vi "Execute.vi"(0 "Session Handle in":T1, 11 "error in (no error)":errorcluster) -> (4 "Session Handle out":T1, 15 "error out":errorcluster)   [LabVIEW 2020, in "TSS.lvlib" / "Execution.lvclass"]
uses:
  Execution.lvclass
  Typedefs/Session Handle.ctl
  Execution.lvclass/Execution.ctl
  VariableContainer/Get Ref Prop.vi
  SequenceFile/Get Ref Prop.vi
  Engine/Get Engine Ref.vi
  SequenceFile/SequenceFile.lvclass
  Engine/Engine.lvclass
  VariableContainer/VariableContainer.lvclass
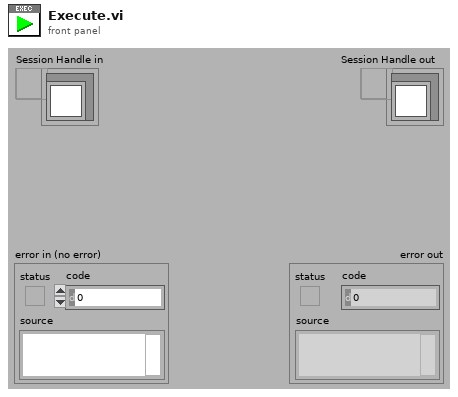
[diagram p1: front panel]
types:
  T1 = typedef "TSS.lvlib/Execution.lvclass/Session Handle.ctl" = refnum<data-value>
  T2 = typedef "TSS.lvlib/Engine.lvclass/Session Handle.ctl" = refnum<data-value>
  T3 = typedef "TSS.lvlib/SequenceFile.lvclass/Session Handle.ctl" = refnum<data-value>
  T4 = typedef "TSS.lvlib/VariableContainer.lvclass/Session Handle.ctl" = refnum<data-value>
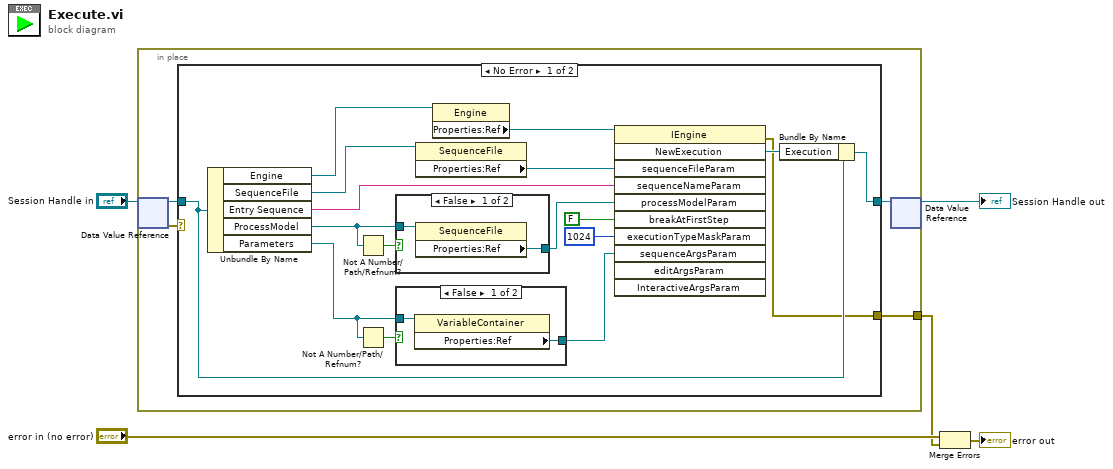
[diagram p0: block diagram]
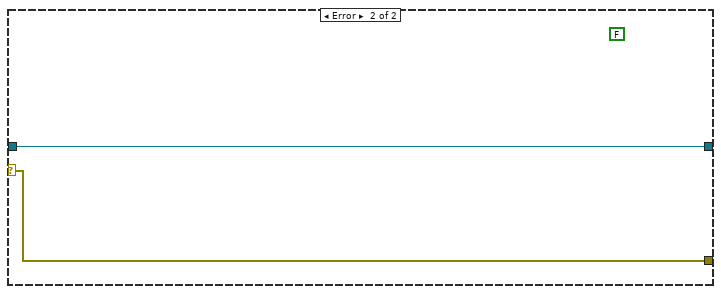
[diagram p4: hidden frame]
diagram:
  n1 = in-place {
    in-place-border: [w6] -> w1
    n2 = in-place-dvr #1("Session Handle in") -> (w9:refnum<class "Execution.lvclass">, w7:errorcluster)
    n3 = case shown="No Error" w7 {
      selector: w7 -> [_ w32]
      tunnel: w9 -> [w14 w31]
      tunnel: [w13 w31] -> w8
      tunnel: [w10 w32] -> w6
      frame No Error {
        n4 = Unbundle By Name(w14) -> ("Engine"=w26:T2, "SequenceFile"=w24:T3, "Entry Sequence"=w22:string, "ProcessModel"=w19:T3, "Parameters"=w16:T4)
        n5 = Not A Number/Path/Refnum?(number/path/refnum=w19) -> (NaN/Path/Refnum?=w20:bool)
        n6 = Not A Number/Path/Refnum?(number/path/refnum=w16) -> (NaN/Path/Refnum?=w17:bool)
        n7 = case shown="False" w20 {
          tunnel: w19 -> [w30 _]
          tunnel: [w29 _] -> w18
          frame False {
            n8 = property class="SequenceFile"(reference=w30) -> ("Properties:Ref"=w29:refnum<k7>)  [unwired: 1 in, 2 out]
          }
          frame True {
          }
        }
        n9 = case shown="False" w17 {
          tunnel: w16 -> [w28 _]
          tunnel: [w27 _] -> w15
          frame False {
            n10 = property class="VariableContainer"(reference=w28) -> ("Properties:Ref"=w27:refnum<k7>)  [unwired: 1 in, 2 out]
          }
          frame True {
          }
        }
        n11 = property class="SequenceFile"(reference=w24) -> ("Properties:Ref"=w23:refnum<k7>)  [unwired: 1 in, 2 out]
        n12 = property class="Engine"(reference=w26) -> ("Properties:Ref"=w25:refnum<k7>)  [unwired: 1 in, 2 out]
        n13 = invoke class="IEngine" method="NewExecution"(reference=w25, "sequenceFileParam"=w23, "sequenceNameParam"=w22, "processModelParam"=w18, "breakAtFirstStep"=FALSE, "executionTypeMaskParam"=1024, "sequenceArgsParam"=w15) -> (error out=w10:errorcluster, "NewExecution"=w11:refnum<k7>)  [unwired: 4 in, 9 out]
        n14 = Bundle By Name(cluster=w14, "Execution"=w11) -> (w13:refnum<class "Execution.lvclass">)
      }
      frame Error {
        (unwired) FALSE ("Auto Release")
      }
    }
    n15 = in-place-dvr #1(w8) -> (→"Session Handle out":T1)  [unwired: 1 out]
  }
  n16 = Merge Errors("error in (no error)", w1) -> (→"error out":errorcluster)
